vi "Compuertas.vi"(9 "FALLA":bool, 10 "CONSOLIDACION":bool, 11 "SATURACION":bool) -> (3 "Boolean":bool)   [LabVIEW 2013]
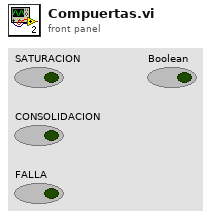
[diagram p1: front panel]
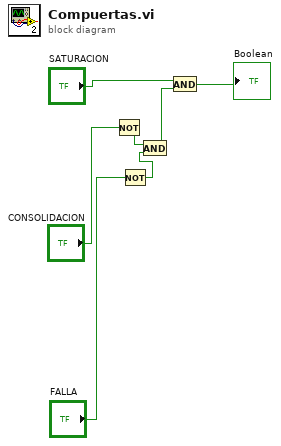
[diagram p0: block diagram]
diagram:
  n1 = Not(x="CONSOLIDACION") -> (.not. x?=w5:bool)
  n2 = Not(x="FALLA") -> (.not. x?=w3:bool)
  n3 = And(x=w5, y=w3) -> (x .and. y?=w6:bool)
  n4 = And(x="SATURACION", y=w6) -> (x .and. y?=→"Boolean":bool)
